vi "Configure Digital Port Pins.vi"(7 "Polarity (0: Voltage High)":i32(ring) items=["Voltage High", "Voltage Low"], 8 "error in (no error)":errorcluster, 9 "Function (0: General Purpose)":i32(ring) items=["General Purpose", "Digital Input-only", "Trigger Output", "Trigger Input", "Isolated Fault Output ", "Inhibit Input", "On Control", "Off Control"], 10 "Pins (1 : Pin 1)":i32(ring)=1 items=["Pin 1"=1, "Pin 2"=2, "Pin 3"=3], 11 "VISA resource name":refnum<visa-resource-name>) -> (0 "error out":errorcluster, 3 "VISA resource name out":refnum<visa-resource-name>)   [LabVIEW 2020, in "Keysight E36300 Series.lvlib"]
doc: "Configures the digital port pins.\n\n<b>Note: </b>\nThis VI is only applicable for E36312A and E36313A models."
uses:
  Keysight E36300 Series.lvlib
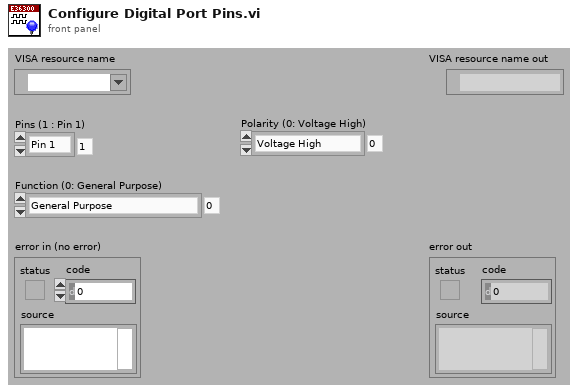
[diagram p1: front panel]
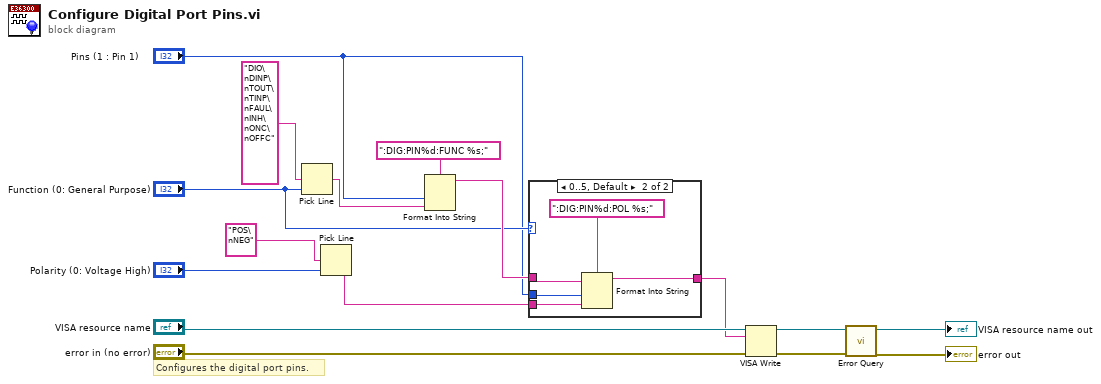
[diagram p0: block diagram]
diagram:
  # "Configures the digital port pins."
  n1 = Pick Line(multi-line string="DIO\nDINP\nTOUT\nTINP\nFAUL\nINH\nONC\nOFFC", line index="Function (0: General Purpose)") -> (output string=w14:string)  [unwired: 1 in]
  n2 = Pick Line(multi-line string="POS\nNEG", line index="Polarity (0: Voltage High)") -> (output string=w4:string)  [unwired: 1 in]
  n3 = Format Into String(format string=":DIG:PIN%d:FUNC %s;", "Pins (1 : Pin 1)", w14) -> (resulting string=w5:string)  [unwired: 2 in, 1 out]
  n4 = case shown="0..5, Default" "Function (0: General Purpose)" {
    tunnel: w5 -> [w17 w22]
    tunnel: "Pins (1 : Pin 1)" -> [_ w21]
    tunnel: w4 -> [_ w20]
    tunnel: [w17 w19] -> w2
    frame 6, 7 {
    }
    frame 0..5, Default {
      n5 = Format Into String(format string=":DIG:PIN%d:POL %s;", initial string=w22, w21, w20) -> (resulting string=w19:string)  [unwired: 1 in, 1 out]
    }
  }
  n6 = VISA Write(VISA resource name="VISA resource name", write buffer=w2, error in (no error)="error in (no error)") -> (VISA resource name out=w9:refnum<visa-resource-name>, error out=w8:errorcluster)  [unwired: 1 out]
  n7 = call "Error Query.vi"("error in (no error)"=w8, "VISA resource name"=w9) -> ("error out"=→"error out":errorcluster, "VISA resource name out"=→"VISA resource name out":refnum<visa-resource-name>)  [unwired: 6 in, 2 out]
